vi "Pitch Marker List.vi"(9 "Number of Octaves":i32, 10 "Input Pitch Enum":T1(array[ring])) -> (2 "Output Freq Array":dbl[](array[numeric]))   [LabVIEW 2012]
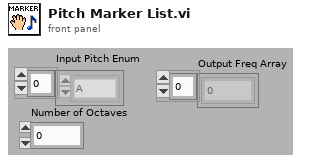
[diagram p1: front panel]
types:
  T1 = enum16{"A", "A#", "B", "C", "C#", "D", "D#", "E", "F", "F#", "G", "G#"}[]
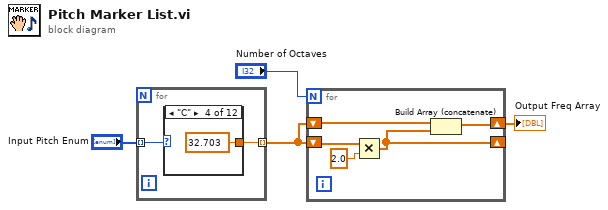
[diagram p0: block diagram]
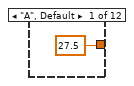
[diagram p2: hidden frame]
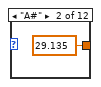
[diagram p3: hidden frame]
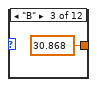
[diagram p4: hidden frame]
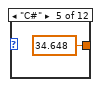
[diagram p5: hidden frame]
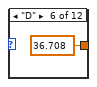
[diagram p6: hidden frame]
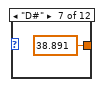
[diagram p7: hidden frame]
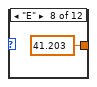
[diagram p8: hidden frame]
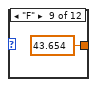
[diagram p9: hidden frame]
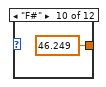
[diagram p10: hidden frame]
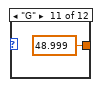
[diagram p11: hidden frame]
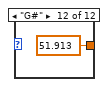
[diagram p12: hidden frame]
diagram:
  n1 = for {
    tunnel: "Input Pitch Enum" -> [w6] mode=indexing
    tunnel: [w5] -> w3 mode=indexing
    n2 = case shown="\"C\"" w6 {
      tunnel: [27.5 29.135 30.868 32.703 34.648 36.708 38.891 41.203 43.654 46.249 48.999 51.913] -> w5
      frame "A", Default {
      }
      frame "A#" {
      }
      frame "B" {
      }
      frame "C" {
      }
      frame "C#" {
      }
      frame "D" {
      }
      frame "D#" {
      }
      frame "E" {
      }
      frame "F" {
      }
      frame "F#" {
      }
      frame "G" {
      }
      frame "G#" {
      }
    }
  }
  n3 = for {
    N: "Number of Octaves" -> [_]
    shift-right: [w19] -> _
    shift-left: w3 -> [w23]
    shift-right: [w20] -> w1
    shift-left: w3 -> [w21]
    n4 = Multiply(x=w23, y=2.0) -> (x*y=w19:dbl[])
    n5 = Build Array (concatenate)(w21, w19) -> (w20:dbl[])
  }
  "Output Freq Array" <- w1
